vi "Threshold Alert.vi"(8 "error in (no error)":errorcluster, 10 "Value":dbl format="%#_13g", 11 "Message":string) -> (0 "error out":errorcluster)   [LabVIEW 2018, in "Testing UI 1.lvlib"]
doc: "This subVI enqueues the named action in to the communications queue along with the input data."
uses:
  Testing UI 1.lvlib
  Private Controls/Module Data.ctl
  Private Controls/Module Action.ctl
panel:
  out "concatenated string":string
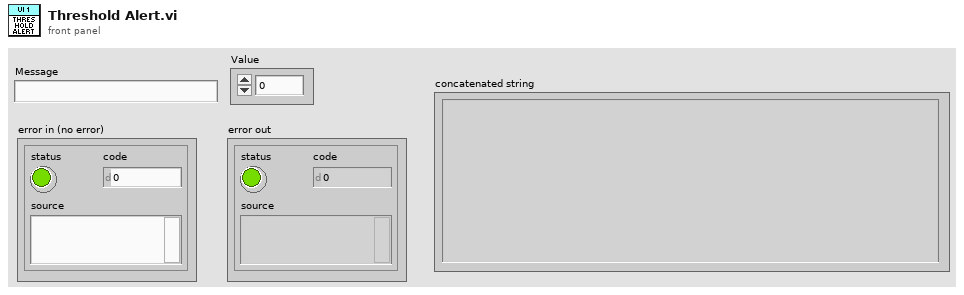
[diagram p1: front panel]
types:
  T1 = typedef "Testing UI 1.lvlib/Module Action.ctl" = enum8{"Init", "Open FP", "Timeout", "New Report Value", "Update Test Info", "Record Data", "Update Report Path", "SetFuelPressure", "Error", "Exit", "Update System Log", "Load APU Setup Data", "Threshold ALERT", "Engine Start Val Change", "Value to Record"}
  T2 = typedef "Testing UI 1.lvlib/Module Data.ctl" = cluster{"Data":variant, "Action":T1}
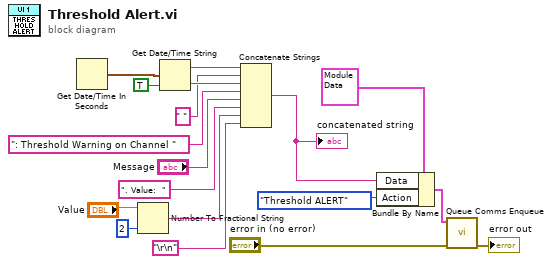
[diagram p0: block diagram]
diagram:
  n1 = Get Date/Time In Seconds() -> (seconds since 1Jan1904=w8:timestamp)
  n2 = Number To Fractional String(number="Value", precision (6)=i16 2) -> (F-format string=w3:string)  [unwired: 2 in]
  n3 = Get Date/Time String(seconds (now)=w8, want seconds? (F)=TRUE) -> (date string=w11:string, time string=w13:string)  [unwired: 1 in]
  n4 = Concatenate Strings(w11, " " ("string"), w13, ": Threshold Warning on Channel " ("string"), "Message", ". Value:  " ("string"), w3, "\r\n") -> (w7:string)
  "concatenated string" <- w7
  n5 = Bundle By Name(cluster=T2 {"Data"=variant, "Action"=enum."Init"} ("element"), "Data"=w7, "Action"=Module_Action."Threshold ALERT") -> (w18:T2)
  n6 = call "Queue Comms Enqueue.vi"("error in (no error)"="error in (no error)", "element"=w18) -> ("error out"=→"error out":errorcluster)  [unwired: 9 in]
